vi "getdVbydt.vi"(9 "times":dbl[](array[numeric]), 11 "voltages":dbl[](array[numeric])) -> (1 "dT":dbl, 2 "dV/dT":dbl, 3 "dV":dbl)   [LabVIEW 2021]
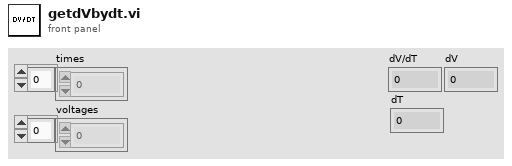
[diagram p1: front panel]
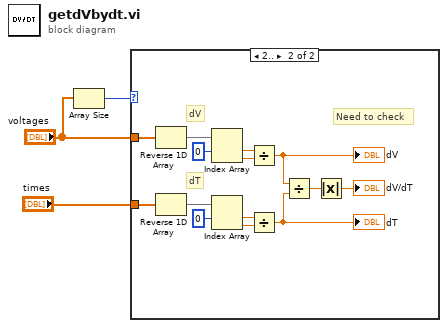
[diagram p0: block diagram]
diagram:
  n1 = Array Size(array="voltages") -> (size(s)=w3:i32)
  n2 = case shown="2.." w3 {
    tunnel: "voltages" -> [_ w17]
    tunnel: "times" -> [_ w8]
    frame ..1 {
    }
    frame 2.. {
      # "Need to check"
      # "dT"
      # "dV"
      n3 = Reverse 1D Array(array=w17) -> (reversed array=w16:dbl[])
      n4 = Reverse 1D Array(array=w8) -> (reversed array=w9:dbl[])
      n5 = Index Array(array=w16, index #1=0 ("index")) -> (element #1=w14:dbl, element #2=w13:dbl)  [unwired: 1 in]
      n6 = Index Array(array=w9, index #1=0 ("index")) -> (element #1=w11:dbl, element #2=w12:dbl)  [unwired: 1 in]
      n7 = Divide(x=w14, y=w13) -> (x/y=w4:dbl)
      "dV" <- w4
      n8 = Divide(x=w11, y=w12) -> (x/y=w5:dbl)
      "dT" <- w5
      n9 = Divide(x=w4, y=w5) -> (x/y=w7:dbl)
      n10 = Absolute Value(x=w7) -> (abs(x)=→"dV/dT":dbl)
    }
  }
